vi "FileIO-Insert Header Data.vi"(0 "path":path, 5 "Header label":string, 9 "Header data":dbl[](array[numeric]), 11 "error in (no error)":errorcluster) -> (15 "error out":errorcluster)   [LabVIEW 2015]
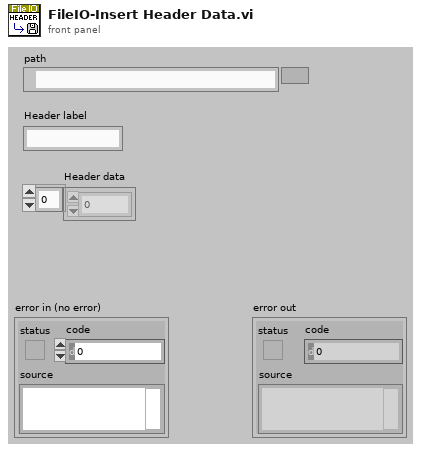
[diagram p1: front panel]
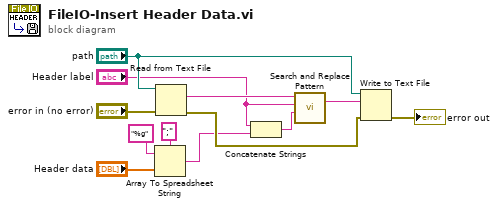
[diagram p0: block diagram]
diagram:
  n1 = Array To Spreadsheet String(delimiter (Tab)=";", array="Header data", 3:"%g" ("format string")) -> (spreadsheet string=w2:string)
  n2 = Read from Text File(file (use dialog)="path", error in="error in (no error)") -> (text=w12:string, error out=w8:errorcluster)  [unwired: 2 in, 2 out]
  n3 = Concatenate Strings("Header label", w2) -> (w11:string)
  n4 = call <vilib>:"Search and Replace Pattern.vi"("string"=w12, "regular expression (\"\")"="Header label", "replace string (\"\")"=w11) -> ("result string"=w9:string)  [unwired: 2 in, 1 out]
  n5 = Write to Text File(file (use dialog)="path", text=w9, error in=w8) -> (error out=→"error out":errorcluster)  [unwired: 1 in, 2 out]
